vi "IntelSignalSet.vi"(1 "CAN64B簇":cluster{"时间(s)":dbl[], "Data64Bits(u64)":u64[]}, 2 "信号格式簇":T1) -> (6 "信号":cluster{"时间(s)":dbl[], "数据":dbl[]})   [LabVIEW 2015]
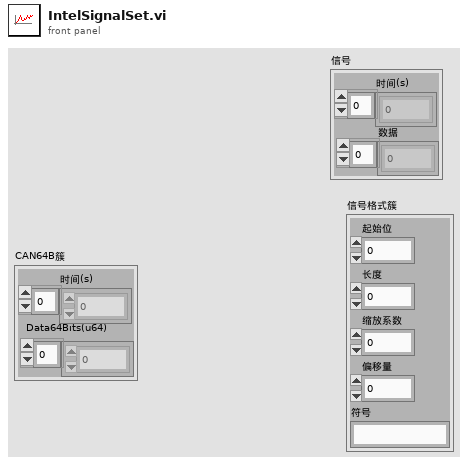
[diagram p1: front panel]
types:
  T1 = cluster{"起始位":u8, "长度":u8, "缩放系数":dbl, "偏移量":dbl, "符号":string}
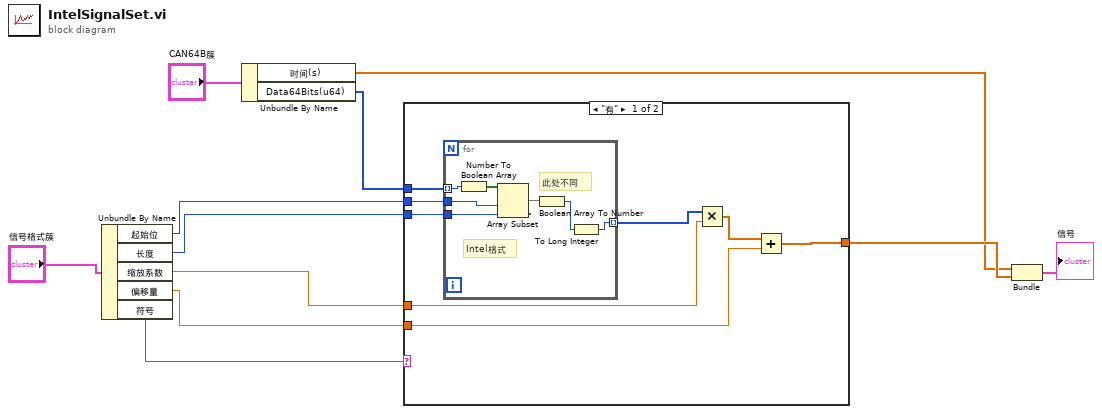
[diagram p0: block diagram]
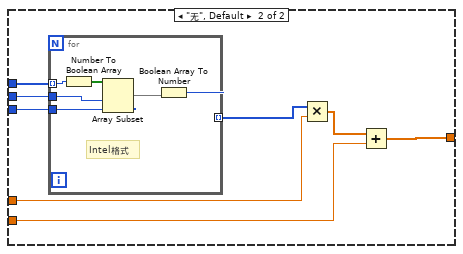
[diagram p2: hidden frame]
diagram:
  n1 = Unbundle By Name("信号格式簇") -> ("起始位"=w5:u8, "长度"=w4:u8, "缩放系数"=w3:dbl, "偏移量"=w2:dbl, "符号"=w1:string)
  n2 = Unbundle By Name("CAN64B簇") -> ("时间(s)"=w7:dbl[], "Data64Bits(u64)"=w8:u64[])
  n3 = case shown="\"有\"" w1 {
    tunnel: [w19 w34] -> w11
    tunnel: w8 -> [w16 w31]
    tunnel: w5 -> [w15 w30]
    tunnel: w4 -> [w14 w29]
    tunnel: w3 -> [w13 w28]
    tunnel: w2 -> [w12 w27]
    frame "有" {
      n4 = for {
        tunnel: w16 -> [w24] mode=indexing
        tunnel: w15 -> [w26]
        tunnel: w14 -> [w25]
        tunnel: [w20] -> w17 mode=indexing
        # "此处不同"
        # "Intel格式"
        n5 = Number To Boolean Array(number=w24) -> (Boolean array=w23:bool[])
        n6 = Array Subset(array=w23, index=w26, length=w25) -> (w22:bool[])
        n7 = Boolean Array To Number(Boolean array=w22) -> (number=w21:u32)
        n8 = To Long Integer(number=w21) -> (32bit integer=w20:i32)
      }
      n9 = Multiply(x=w17, y=w13) -> (x*y=w18:dbl[])
      n10 = Add(x=w18, y=w12) -> (x+y=w19:dbl[])
    }
    frame "无", Default {
      n11 = for {
        tunnel: w31 -> [w37] mode=indexing
        tunnel: w30 -> [w40]
        tunnel: w29 -> [w39]
        tunnel: [w38] -> w32 mode=indexing
        # "Intel格式"
        n12 = Number To Boolean Array(number=w37) -> (Boolean array=w36:bool[])
        n13 = Array Subset(array=w36, index=w40, length=w39) -> (w35:bool[])
        n14 = Boolean Array To Number(Boolean array=w35) -> (number=w38:u32)
      }
      n15 = Multiply(x=w32, y=w28) -> (x*y=w33:dbl[])
      n16 = Add(x=w33, y=w27) -> (x+y=w34:dbl[])
    }
  }
  n17 = Bundle("时间(s)"=w7, w11) -> (→"信号":cluster{"时间(s)":dbl[], dbl[]})  [unwired: 1 in]
